vi "Value.vi"(8 "error in (no error)":errorcluster, 11 "ColumnPanel in":refnum<class "ColumnPanel.lvclass">) -> (0 "error out":errorcluster, 2 "Type Value":refnum<class "Type.lvclass">)   [LabVIEW 2020, in "Conditum-Tools.lvlib" / "ColumnPanel.lvclass"]
uses:
  ColumnPanel.lvclass
  ColumnPanel.lvclass/ColumnPanel.ctl
  Conditum/Columns/Type/Type.lvclass
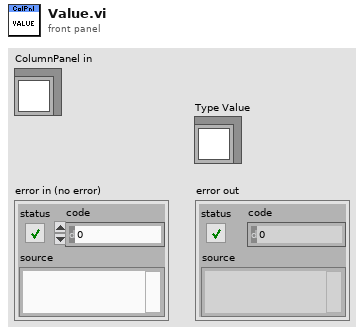
[diagram p1: front panel]
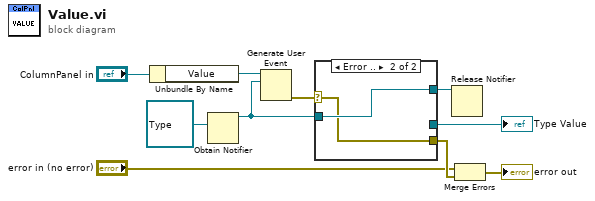
[diagram p0: block diagram]
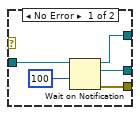
[diagram p2: hidden frame]
diagram:
  n1 = Unbundle By Name("ColumnPanel in") -> ("Value"=w8:refnum<user-event>)
  n2 = Obtain Notifier(notification data type=refnum<class "Type.lvclass"> refnum ("Conditum:Columns:Type.lvclass")) -> (notifier out=w7:refnum<notifier>)  [unwired: 3 in, 2 out]
  n3 = Generate User Event(user event=w8, event data cluster=w7) -> (error out=w6:errorcluster)  [unwired: 2 in, 1 out]
  n4 = case shown="Error .." w6 {
    selector: w6 -> [_ w16]
    tunnel: w7 -> [w15 w17]
    tunnel: [w13 _] -> w5
    tunnel: [w12 w17] -> w4
    tunnel: [w11 w16] -> w3
    frame No Error {
      n5 = Wait on Notification(notifier=w15, timeout in ms (-1)=100) -> (notifier out=w12:refnum<notifier>, notification=w13:refnum<class "Type.lvclass">, error out=w11:errorcluster)  [unwired: 2 in, 1 out]
    }
    frame Error {
    }
  }
  "Type Value" <- w5
  n6 = Release Notifier(notifier=w4) -> ()  [unwired: 2 in, 3 out]
  n7 = Merge Errors("error in (no error)", w3) -> (→"error out":errorcluster)
